vi "PH_Cont-601k_PSU.destructor.vi"(0 "i ref in":refnum<vi>, 5 "error in(no error)":errorcluster) -> (19 "error out":errorcluster)   [LabVIEW 2014, in "PH_Cont-601k_PSU.lvlib"]
doc: "This is the destructor of a class.\n\nLicense Agreement for this software:\n\nCopyright (C)\nGesellschaft für Schwerionenforschung, GSI\nPlanckstr. 1\n64291 Darmstadt\nGermany\n\nContact: D.Beck@gsi.de \n\nThis program is free software; you can redistribute it and/or modify it under the terms of the \nGNU General Public License as published by the Free Software Foundation; either version 2 of \nthe license, or (at your option) any later version.\n\nThis program is distributed in the hope that it will be useful, but WITHOUT ANY WARRANTY; \nwithout even the implied warranty of MERCHANTABILITY or FITNESS FOR A PARTICULAR PURPOSE. See the GNU General License for more details (http://www.gnu.org).\n\nGesellschaft für Schwerionenforschung, GSI\nPlanckstr. 1, 64291 Darmstadt, Germany\nFor all questions and ideas contact: M.Richter@gsi.de, H.Brand@gsi.de or D.Beck@gsi.de.\nLast update: 16-JUN-2004"
uses:
  PH_Cont-601k_PSU.lvlib
  PH_Cont-601k_PSU.Readyness.ctl
  PH_Cont-601k_PSU.Readyness Program.ctl
  PH_Cont-601k_PSU.Readyness Device.ctl
  lib.lib/DimLVEvent/LVDimInterface/LVDimInterface.lvlib
  non_GPL/instr.lib/pu601k/Continuum PU610K - Driver np.lvlib
  PH_Class/PH_Class.lvlib
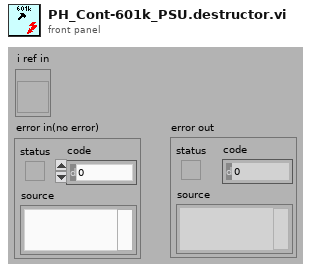
[diagram p1: front panel]
types:
  T1 = typedef "PH_Cont-601k_PSU.lvlib/PH_Cont-601k_PSU.i attribute.ctl" = cluster{"GUI Refs":T2, "Interlock":bool, "Service ID applied Voltage":i32, "Device Settings":cluster{"Configuration":T3, "Flash Interval [s]":dbl, "Mode":T4, "Voltage [V]":u16, "Charge":bool, "VISA resource name":refnum<visa-resource-name>}, "Readyness":T5, "Information":cluster{"VISA resource name":refnum<visa-resource-name>, "Tagname Power On":string, "Interlock":cluster{"Instance":string, "Tagname":string}, "Limits [V]":cluster{"Lower":dbl, "Upper":dbl}, "Tagname PSU On":string}, "R2S":bool, "Charge is allowed":bool}
  T2 = typedef "PH_Cont-601k_PSU.lvlib/PH_Cont-601k_PSU.GUI Refs.ctl" = cluster{"Power On":refnum<vi>, "Hard- and Software":refnum<vi>, "Device Status":refnum<vi>, "Device Error":refnum<vi>, "Configuration":refnum<vi>, "Flash Interval [s]":refnum<vi>, "Interlock":refnum<vi>, "Interlock Indicator":refnum<vi>, "Voltage [V]":refnum<vi>, "Readyness":refnum<vi>, "Mode":refnum<vi>, "Reset Error":refnum<vi>, "Expert working":refnum<vi>, "Charge":refnum<vi>, "PSU On":refnum<vi>}
  T3 = typedef "PH_Cont-601k_PSU.lvlib/PH_Cont-601k_PSU.Configuration.ctl" = u16
  T4 = typedef "PH_Cont-601k_PSU.lvlib/PH_Cont-601k_PSU.Mode.ctl" = enum32{"STOP", "STANDBY", "READY", "EMISSION", "ERROR"}
  T5 = typedef "PH_Cont-601k_PSU.lvlib/PH_Cont-601k_PSU.Readyness.ctl" = cluster{"Program":T6, "Device":T7}
  T6 = typedef "PH_Cont-601k_PSU.lvlib/PH_Cont-601k_PSU.Readyness Program.ctl" = enum32{"OFF", "POWER", "INTERLOCK"}
  T7 = typedef "PH_Cont-601k_PSU.lvlib/PH_Cont-601k_PSU.Readyness Device.ctl" = enum32{"OFF", "CONNECTING", "CONNECTED", "OPERATING", "EOC", "ERROR"}
  T8 = enum16{"SetAttribute", "GetAttribute", "CreateAttribute", "DestroyAttribute", "DestroyAllAtributes"}
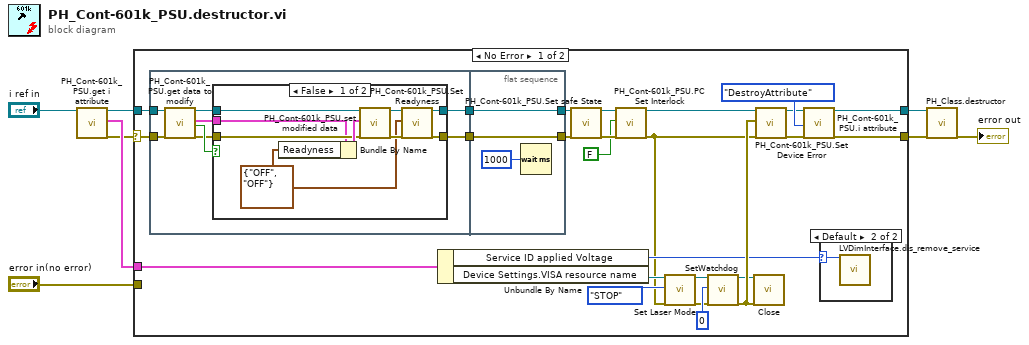
[diagram p0: block diagram]
diagram:
  n1 = call "PH_Cont-601k_PSU.get i attribute.vi"("i ref in"="i ref in") -> ("i ref out"=w4:refnum<vi>, "i attribute"=w7:T1, "error out"=w3:errorcluster)  [unwired: 16 in]
  n2 = case shown="No Error" w3 {
    selector: w3 -> [w9 _]
    tunnel: [w31 w58] -> w8
    tunnel: w7 -> [w30 _]
    tunnel: [w29 w57] -> w6
    tunnel: w4 -> [w10 w57]
    tunnel: "error in(no error)" -> [_ w58]
    frame No Error {
      n3 = flat-sequence {
        tunnel: w10 -> [w40]
        tunnel: w9 -> [w39]
        tunnel: [w42] -> w33
        tunnel: [w41] -> w32
        tunnel: [w55] -> w27
        tunnel: [w56] -> w26
        tunnel: w33 -> [w56]
        tunnel: w32 -> [w55]
        frame #0 {
          n4 = call "PH_Cont-601k_PSU.get data to modify.vi"("i ref in"=w40, "error in (no error)"=w39) -> ("i ref out"=w38:refnum<vi>, "i attribute"=w37:T1, "timed out"=w36:bool, "error out"=w35:errorcluster)  [unwired: 14 in]
          n5 = case shown="False" w36 {
            tunnel: w38 -> [w51 w53]
            tunnel: w37 -> [w43 _]
            tunnel: [w48 w53] -> w42
            tunnel: [w46 w52] -> w41
            tunnel: w35 -> [w45 w52]
            frame False {
              w44 = T5 {"Program"=enum."OFF", "Device"=enum."OFF"} ("Readyness")
              n6 = Bundle By Name(cluster=w43, "Readyness"=w44) -> (w50:T1)
              n7 = call "PH_Cont-601k_PSU.set modified data.vi"("i ref in"=w51, "i attribute"=w50, "error in (no error)"=w45) -> ("i ref out"=w49:refnum<vi>, "error out"=w47:errorcluster)  [unwired: 15 in]
              n8 = call "PH_Cont-601k_PSU.Set Readyness.vi"("VI in"=w49, "Current Readyness"=w44, "error in (no error)"=w47) -> ("VI out"=w48:refnum<vi>, "error out"=w46:errorcluster)  [unwired: 15 in]
            }
            frame True {
            }
          }
        }
        frame #1 {
          n9 = Wait (ms)(milliseconds to wait=u32 1000) -> ()  [unwired: 1 out]
        }
      }
      n10 = Unbundle By Name(w30) -> ("Service ID applied Voltage"=w15:i32, "Device Settings.VISA resource name"=w20:refnum<visa-resource-name>)
      n11 = call "PH_Cont-601k_PSU.Set safe State.vi"("VI in"=w26, "error in (no error)"=w27) -> ("VI out"=w17:refnum<vi>, "error out"=w21:errorcluster)  [unwired: 16 in]
      n12 = call "PH_Cont-601k_PSU.PC Set Interlock.vi"("VI in"=w17, "Set Interlock"=FALSE, "error in (no error)"=w21) -> ("VI out"=w12:refnum<vi>, "error out"=w11:errorcluster)  [unwired: 15 in]
      n13 = call "Set Laser Mode.vi"("VISA resource name"=w20, "Mode"=enum16{"STOP", "STANDBY", "READY", "EMISSION"}."STOP", "error in"=w11) -> ("VISA resource name out"=w23:refnum<visa-resource-name>, "error out"=w22:errorcluster)  [unwired: 15 in]
      n14 = call "SetWatchdog.vi"("VISA resource name"=w23, "watchdog time (1s)"=u16 0 ("watchdog time (s)"), "error in"=w22) -> ("VISA resource name out"=w18:refnum<visa-resource-name>, "error out"=w19:errorcluster)  [unwired: 15 in]
      n15 = call "Close.vi"("VISA resource name"=w18, "error in (no error)"=w19) -> ()  [unwired: 17 in, 1 out]
      n16 = call "PH_Cont-601k_PSU.Set Device Error.vi"("VI in"=w12, "Device Error"=w19, "error in (no error)"=w11) -> ("VI out"=w14:refnum<vi>, "error out"=w13:errorcluster)  [unwired: 15 in]
      n17 = call "PH_Cont-601k_PSU.i attribute.vi"("VI Refnum"=w14, "Action"=T8."DestroyAttribute", "error in (no error)"=w13) -> ("VI Refnum out"=w29:refnum<vi>, "error out"=w31:errorcluster)  [unwired: 14 in, 1 out]
      n18 = case shown="Default" w15 {
        selector: w15 -> [_ w34]
        frame -1 {
        }
        frame Default {
          n19 = call "LVDimInterface.dis_remove_service.vi"("my_serviceID"=w34) -> ()  [unwired: 18 in, 1 out]
        }
      }
    }
    frame Error {
    }
  }
  n20 = call "PH_Class.destructor.vi"("i ref in"=w6, "error in(no error)"=w8) -> ("error out"=→"error out":errorcluster)  [unwired: 17 in]
